vi "OLA.vi"() -> ()   [LabVIEW 2010]
doc: "This is the On-Line Analysis module (OLA).\nThis module receives events from the Target Event Builder (TEB) and processes them. The Q Curve is massaged, gains are divided out, the subtracted and poly subtracted signals are calculated, and an area measurement is made. These results are then sent to the Polarization Display Panel (PDP)."
panel:
  out "Bottom Charge":dbl format="%.6e"
  out "Top Charge":dbl format="%.6e"
  in  "Previous Event":i32
  in  "stop":bool
  out "RF Mod":i32
  out "RF Freq":dbl format="%.3f"
  out "Cal Const":dbl format="%.6f"
  out "Baseline":i32
  out "Raw Signal":dbl[](array[numeric]) format="%.4f"
  out "Event Number":i32
  out "Area":dbl format="%.6f"
  out "Polarization":dbl format="%.2f"
  out "PolySubtracted Signal":dbl[](array[numeric]) format="%.4f"
  out "Polyfit Curve":dbl[](array[numeric]) format="%.4f"
  out "Subtracted Signal":dbl[](array[numeric]) format="%.4f"
  out "Baseline Signal":dbl[](array[numeric]) format="%.6f"
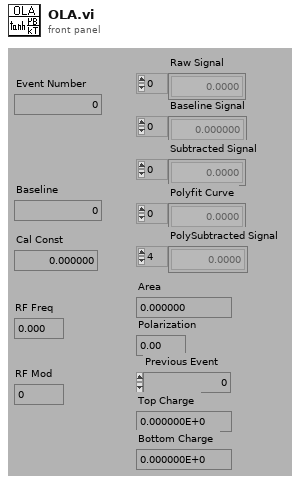
[diagram p1: front panel]
types:
  T1 = enum16{"No Message", "Bad Message", "ClearCharge", "Event=", "Address=", "Ping=", "Stop"}
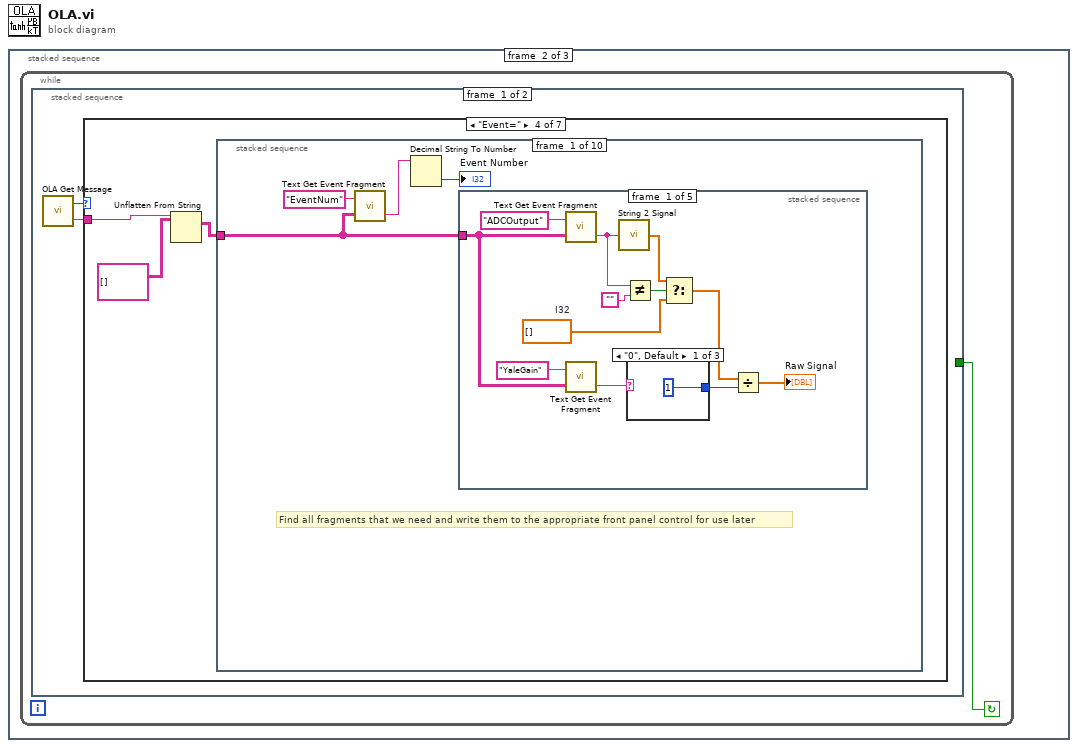
[diagram p0: block diagram]
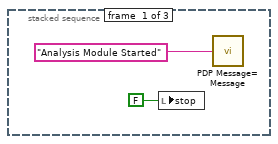
[diagram p2: hidden frame]
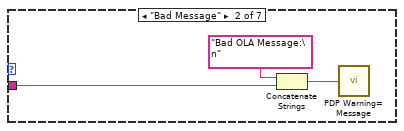
[diagram p4: hidden frame]
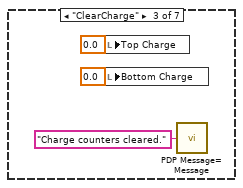
[diagram p5: hidden frame]
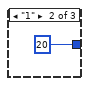
[diagram p6: hidden frame]
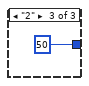
[diagram p7: hidden frame]
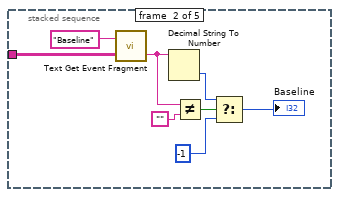
[diagram p8: hidden frame]
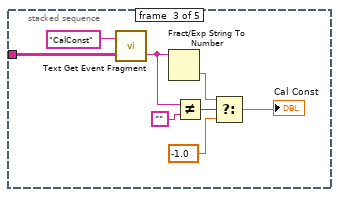
[diagram p9: hidden frame]
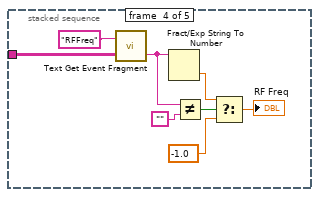
[diagram p10: hidden frame]
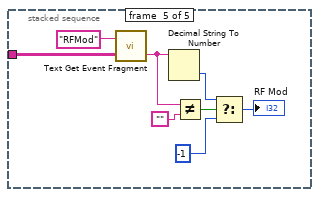
[diagram p11: hidden frame]
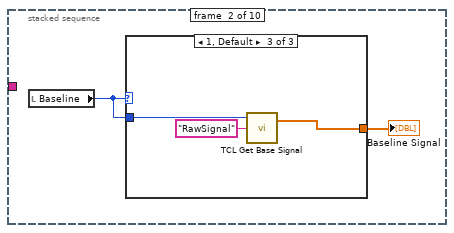
[diagram p12: hidden frame]
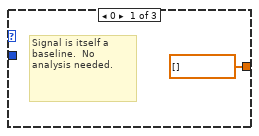
[diagram p13: hidden frame]
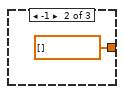
[diagram p14: hidden frame]
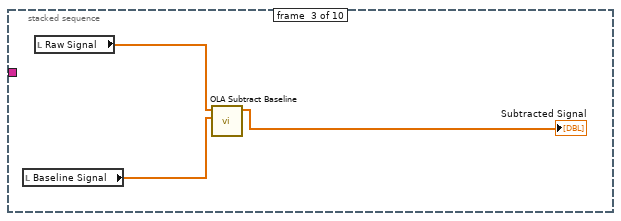
[diagram p15: hidden frame]
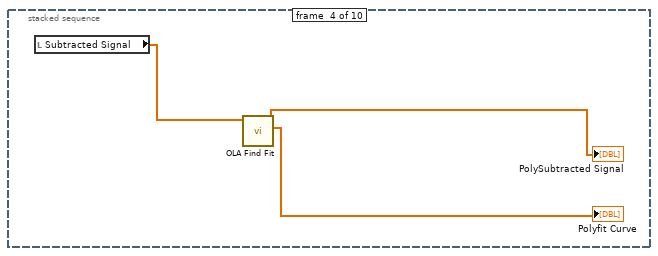
[diagram p16: hidden frame]
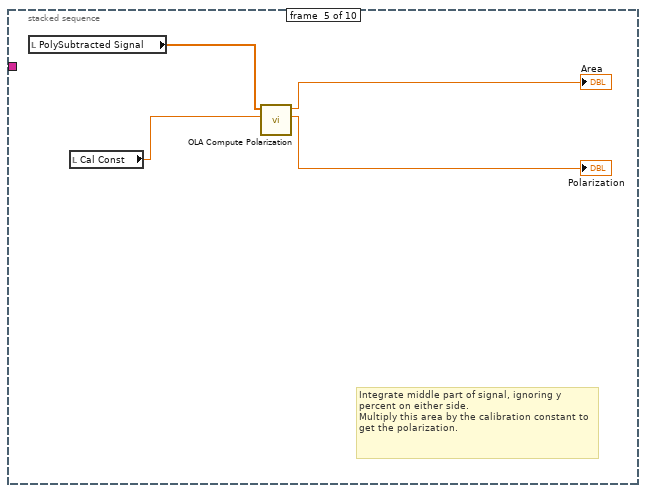
[diagram p17: hidden frame]
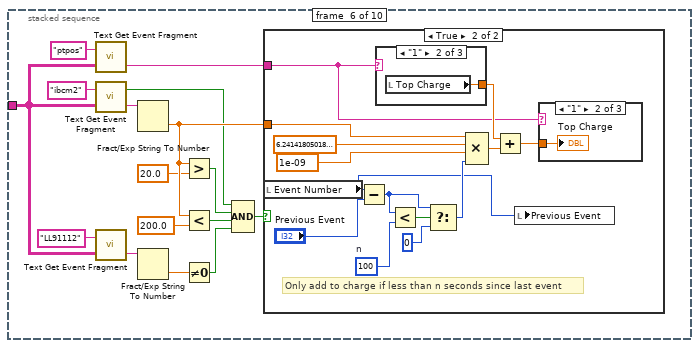
[diagram p18: hidden frame]
diagram:
  n1 = stacked-sequence {
    frame #0 {
      n2 = local write "stop"(FALSE ("stop")) -> ()
      n3 = call "PDP Message= Message.vi"("Message"="Analysis Module Started") -> ()
    }
    frame #1 {
      n4 = while {
        stop <- w3 continue-if-true
        n5 = stacked-sequence {
          tunnel: [_ w221] -> w3
          frame #0 {
            n6 = call "OLA Get Message.vi"() -> ("Text"=w5:string, "OLA Message Type"=w4:T1)
            n7 = case shown="\"Event=\"" w4 {
              tunnel: w5 -> [_ w8 _ w13 w213 w216 _]
              frame "No Message" {
              }
              frame "Bad Message" {
                n8 = Concatenate Strings("Bad OLA Message:\n", w8) -> (w6:string)
                n9 = call "PDP Warning= Message.vi"("Message"=w6) -> ()
              }
              frame "ClearCharge" {
                n10 = local write "Top Charge"(0.0 ("Top Charge")) -> ()
                n11 = local write "Bottom Charge"(0.0 ("Bottom Charge")) -> ()
                n12 = call "PDP Message= Message.vi"("Message"="Charge counters cleared.") -> ()
              }
              frame "Event=" {
                (unwired) FALSE
                n13 = Unflatten From String(type=string[][] [], binary string=w13) -> (value=w12:string[][])  [unwired: 3 in, 2 out]
                n14 = stacked-sequence {
                  tunnel: w12 -> [w15 _ _ _ _ w86 w119 w138 _ _]
                  frame #0 {
                    # "Find all fragments that we need and write them to the appropriate front panel control for use later"
                    n15 = call "Text Get Event Fragment.vi"("Event"=w15, "Fragment Type"="EventNum") -> ("Fragment"=w17:string)  [unwired: 1 out]
                    n16 = Decimal String To Number(string=w17) -> (number=→"Event Number":i32)  [unwired: 2 in, 1 out]
                    n17 = stacked-sequence {
                      tunnel: w15 -> [w24 w40 w48 w56 w64]
                      frame #0 {
                        w19 = dbl[] []  # I32
                        n18 = call "Text Get Event Fragment.vi"("Event"=w24, "Fragment Type"="ADCOutput") -> ("Fragment"=w29:string)  [unwired: 1 out]
                        n19 = call "Text Get Event Fragment.vi"("Event"=w24, "Fragment Type"="YaleGain") -> ("Fragment"=w23:string)  [unwired: 1 out]
                        n20 = call "String 2 Signal.vi"("String"=w29) -> ("Signal"=w26:dbl[])
                        n21 = Not Equal?(x=w29, y="") -> (x != y?=w28:bool)
                        n22 = case shown="\"0\", Default" w23 {
                          tunnel: [1 20 50] -> w22
                          frame "0", Default {
                          }
                          frame "1" {
                          }
                          frame "2" {
                          }
                        }
                        n23 = Select(t=w26, s=w28, f=w19) -> (s? t:f=w21:dbl[])
                        n24 = Divide(x=w21, y=w22) -> (x/y=→"Raw Signal":dbl[])
                      }
                      frame #1 {
                        n25 = call "Text Get Event Fragment.vi"("Event"=w40, "Fragment Type"="Baseline") -> ("Fragment"=w35:string)  [unwired: 1 out]
                        n26 = Decimal String To Number(string=w35) -> (number=w38:i32)  [unwired: 2 in, 1 out]
                        n27 = Not Equal?(x=w35, y="") -> (x != y?=w37:bool)
                        n28 = Select(t=w38, s=w37, f=-1) -> (s? t:f=→"Baseline":i32)
                      }
                      frame #2 {
                        n29 = call "Text Get Event Fragment.vi"("Event"=w48, "Fragment Type"="CalConst") -> ("Fragment"=w43:string)  [unwired: 1 out]
                        n30 = Fract/Exp String To Number(string=w43) -> (number=w46:dbl)  [unwired: 3 in, 1 out]
                        n31 = Not Equal?(x=w43, y="") -> (x != y?=w45:bool)
                        n32 = Select(t=w46, s=w45, f=-1.0) -> (s? t:f=→"Cal Const":dbl)
                      }
                      frame #3 {
                        n33 = call "Text Get Event Fragment.vi"("Event"=w56, "Fragment Type"="RFFreq") -> ("Fragment"=w51:string)  [unwired: 1 out]
                        n34 = Fract/Exp String To Number(string=w51) -> (number=w54:dbl)  [unwired: 3 in, 1 out]
                        n35 = Not Equal?(x=w51, y="") -> (x != y?=w53:bool)
                        n36 = Select(t=w54, s=w53, f=-1.0) -> (s? t:f=→"RF Freq":dbl)
                      }
                      frame #4 {
                        n37 = call "Text Get Event Fragment.vi"("Event"=w64, "Fragment Type"="RFMod") -> ("Fragment"=w59:string)  [unwired: 1 out]
                        n38 = Decimal String To Number(string=w59) -> (number=w62:i32)  [unwired: 2 in, 1 out]
                        n39 = Not Equal?(x=w59, y="") -> (x != y?=w61:bool)
                        n40 = Select(t=w62, s=w61, f=-1) -> (s? t:f=→"RF Mod":i32)
                      }
                    }
                  }
                  frame #1 {
                    n41 = local read "Baseline"() -> (w67:i32)
                    n42 = case shown="1, Default" w67 {
                      tunnel: w67 -> [_ _ w72]
                      tunnel: [dbl[] [] ("Baseline") dbl[] [] ("Baseline") w71] -> w66
                      frame 0 {
                        # "Signal is itself a baseline.  No analysis needed."
                      }
                      frame -1 {
                      }
                      frame 1, Default {
                        n43 = call "TCL Get Base Signal.vi"("signal name"="RawSignal", "event number"=w72) -> ("signal"=w71:dbl[])  [unwired: 1 in, 1 out]
                      }
                    }
                    "Baseline Signal" <- w66
                  }
                  frame #2 {
                    n44 = local read "Baseline Signal"() -> (w74:dbl[])
                    n45 = local read "Raw Signal"() -> (w75:dbl[])
                    n46 = call "OLA Subtract Baseline.vi"("baseline"=w74, "raw"=w75) -> ("subtracted"=→"Subtracted Signal":dbl[])  [unwired: 9 in]
                  }
                  frame #3 {
                    n47 = local read "Subtracted Signal"() -> (w78:dbl[])
                    n48 = call "OLA Find Fit.vi"("signal"=w78) -> ("fit"=→"Polyfit Curve":dbl[], "subtracted"=→"PolySubtracted Signal":dbl[])  [unwired: 8 in, 1 out]
                  }
                  frame #4 {
                    # "Integrate middle part of signal, ignoring y percent on either side.\nMultiply this area by the calibration constant to get the polarization."
                    n49 = local read "PolySubtracted Signal"() -> (w82:dbl[])
                    n50 = local read "Cal Const"() -> (w81:dbl)
                    n51 = call "OLA Compute Polarization.vi"("cal"=w81, "signal"=w82) -> ("polarization"=→"Polarization":dbl, "area"=→"Area":dbl)  [unwired: 8 in]
                  }
                  frame #5 {
                    n52 = call "Text Get Event Fragment.vi"("Event"=w86, "Fragment Type"="ptpos") -> ("Fragment"=w84:string)  [unwired: 1 out]
                    n53 = call "Text Get Event Fragment.vi"("Event"=w86, "Fragment Type"="ibcm2") -> ("Fragment"=w95:string, "Found"=w83:bool)
                    n54 = call "Text Get Event Fragment.vi"("Event"=w86, "Fragment Type"="LL91112") -> ("Fragment"=w97:string)  [unwired: 1 out]
                    n55 = Fract/Exp String To Number(string=w95) -> (number=w94:dbl)  [unwired: 3 in, 1 out]
                    n56 = Fract/Exp String To Number(string=w97) -> (number=w96:dbl)  [unwired: 3 in, 1 out]
                    n57 = Greater?(x=w94, y=20.0) -> (0:w89:bool)
                    n58 = Less?(x=w94, y=200.0) -> (x < y?=w91:bool)
                    n59 = Not Equal To 0?(x=w96) -> (x != 0?=w90:bool)
                    n60 = Compound Arithmetic op=AND(w83, w89, w91, w90) -> (w88:bool)
                    n61 = case shown="True" w88 {
                      tunnel: w94 -> [_ w109]
                      tunnel: w84 -> [_ w100]
                      frame False {
                      }
                      frame True {
                        w108 = 100  # n
                        # "Only add to charge if less than n seconds since last event"
                        n62 = local read "Event Number"() -> (w99:i32)
                        n63 = Subtract(x=w99, y="Previous Event") -> (x-y=w105:i32)
                        n64 = case shown="\"1\"" w100 {
                          tunnel: [0.0 w116 w117] -> w102
                          frame "0", Default {
                          }
                          frame "1" {
                            n65 = local read "Top Charge"() -> (w116:dbl)
                          }
                          frame "2" {
                            n66 = local read "Bottom Charge"() -> (w117:dbl)
                          }
                        }
                        n67 = Less?(x=w105, y=w108) -> (x < y?=w106:bool)
                        n68 = Select(t=w105, s=w106, f=0) -> (s? t:f=w103:i32)
                        n69 = Compound Arithmetic op=MULTIPLY(w109, 6.241418050181001e+18, 1e-09 ("Input"), w103) -> (w107:dbl)
                        n70 = Add(x=w102, y=w107) -> (x+y=w101:dbl)
                        n71 = local write "Previous Event"(w99) -> ()
                        n72 = case shown="\"1\"" w100 {
                          tunnel: w101 -> [_ w113 w114]
                          frame "0", Default {
                          }
                          frame "1" {
                            "Top Charge" <- w113
                          }
                          frame "2" {
                            "Bottom Charge" <- w114
                          }
                        }
                      }
                    }
                  }
                  frame #6 {
                    n73 = call "Text Get Event Fragment.vi"("Event"=w119, "Fragment Type"="He4Temp") -> ("Found"=w118:bool)  [unwired: 1 out]
                    n74 = case shown="False" w118 {
                      tunnel: w119 -> [w127 _]
                      frame False {
                        n75 = call "Text Get Event Fragment.vi"("Event"=w127, "Fragment Type"="He4Press") -> ("Fragment"=w135:string)  [unwired: 1 out]
                        n76 = call "Text Get Event Fragment.vi"("Event"=w127, "Fragment Type"="He4Range") -> ("Fragment"=w126:string)  [unwired: 1 out]
                        n77 = Fract/Exp String To Number(string=w135) -> (number=w121:dbl)  [unwired: 3 in, 1 out]
                        n78 = Fract/Exp String To Number(string=w126) -> (number=w125:dbl)  [unwired: 3 in, 1 out]
                        n79 = expression code="10**(-x+2)"(w125) -> (w124:dbl)
                        n80 = Multiply(x=w121, y=w124) -> (x*y=w122:dbl)
                        n81 = call "TTM 4He Press to Temp.vi"("4He Vapor Pressure (torr)"=w122) -> ("4He Temp (K)"=w123:dbl)
                        n82 = Number To Exponential String(number=w123) -> (E-format string=w133:string)  [unwired: 3 in]
                        n83 = local read "Event Number"() -> (w130:i32)
                        n84 = Build Array("He4Temp", w133) -> (w129:string[])
                        n85 = Build Array(w129) -> (w131:string[][])
                        n86 = call "TEB EventFrag= Message.vi"("Event Fragment(s)"=w131, "Event Number"=w130) -> ()
                      }
                      frame True {
                      }
                    }
                  }
                  frame #7 {
                    n87 = call "Text Get Event Fragment.vi"("Event"=w138, "Fragment Type"="HPFreq") -> ("Fragment"=w136:string, "Found"=w137:bool)
                    n88 = case shown="True" w137 {
                      tunnel: w138 -> [w141 w159]
                      tunnel: w136 -> [_ w156]
                      frame False {
                        n89 = call "Text Get Event Fragment.vi"("Event"=w141, "Fragment Type"="EIPFreq") -> ("Fragment"=w140:string)  [unwired: 1 out]
                        n90 = local read "Event Number"() -> (w143:i32)
                        n91 = Build Array("uWaveFreq", w140) -> (w142:string[])
                        n92 = Build Array(w142) -> (w144:string[][])
                        n93 = call "TEB EventFrag= Message.vi"("Event Fragment(s)"=w144, "Event Number"=w143) -> ()
                      }
                      frame True {
                        n94 = call "Text Get Event Fragment.vi"("Event"=w159, "Fragment Type"="EIPFreq") -> ("Fragment"=w158:string)  [unwired: 1 out]
                        n95 = Fract/Exp String To Number(string=w156) -> (number=w149:dbl)  [unwired: 3 in, 1 out]
                        n96 = Fract/Exp String To Number(string=w158) -> (number=w157:dbl)  [unwired: 3 in, 1 out]
                        n97 = Multiply(x=w157, y=2) -> (x*y=w155:dbl)
                        n98 = Add(x=w149, y=w155) -> (x+y=w154:dbl)
                        n99 = Equal To 0?(x=w149) -> (x = 0?=w148:bool)
                        n100 = Number To Fractional String(number=w154, precision (6)=i16 3) -> (F-format string=w150:string)  [unwired: 2 in]
                        n101 = Select(t="0", s=w148, f=w150) -> (s? t:f=w151:string)
                        n102 = local read "Event Number"() -> (w161:i32)
                        n103 = Build Array("uWaveFreq", w151) -> (w160:string[])
                        n104 = Build Array(w160) -> (w162:string[][])
                        n105 = call "TEB EventFrag= Message.vi"("Event Fragment(s)"=w162, "Event Number"=w161) -> ()
                      }
                    }
                  }
                  frame #8 {
                    w167 = string[] [] ("Array Constant")
                    # "Ship all results off to the event builder."
                    n106 = local read "PolySubtracted Signal"() -> (w165:dbl[])
                    n107 = local read "Bottom Charge"() -> (w177:dbl)
                    n108 = local read "Subtracted Signal"() -> (w202:dbl[])
                    n109 = local read "Polyfit Curve"() -> (w201:dbl[])
                    n110 = local read "Polarization"() -> (w188:dbl)
                    n111 = local read "Baseline Signal"() -> (w207:dbl[])
                    n112 = local read "Top Charge"() -> (w178:dbl)
                    n113 = local read "Raw Signal"() -> (w185:dbl[])
                    n114 = local read "Area"() -> (w196:dbl)
                    n115 = Array Size(array=w165) -> (size(s)=w166:i32)
                    n116 = Equal To 0?(x=w166) -> (x = 0?=w168:bool)
                    n117 = call "Signal 2 String.vi"("Signal"=w185) -> ("String"=w186:string)
                    n118 = call "Signal 2 String.vi"("Signal"=w207) -> ("String"=w206:string)
                    n119 = call "Signal 2 String.vi"("Signal"=w202) -> ("String"=w203:string)
                    n120 = call "Signal 2 String.vi"("Signal"=w201) -> ("String"=w200:string)
                    n121 = call "Signal 2 String.vi"("Signal"=w165) -> ("String"=w197:string)
                    n122 = Number To Exponential String(number=w178) -> (E-format string=w180:string)  [unwired: 3 in]
                    n123 = Number To Exponential String(number=w177) -> (E-format string=w175:string)  [unwired: 3 in]
                    n124 = Number To Exponential String(number=w188) -> (E-format string=w189:string)  [unwired: 3 in]
                    n125 = Number To Exponential String(number=w196) -> (E-format string=w195:string)  [unwired: 3 in]
                    n126 = Build Array("RawSignal", w186) -> (w184:string[])
                    n127 = Build Array("BaseSignal", w206) -> (w183:string[])
                    n128 = Build Array("SubSignal", w203) -> (w182:string[])
                    n129 = Build Array("PolyCurve", w200) -> (w181:string[])
                    n130 = Build Array("PolySignal", w197) -> (w193:string[])
                    n131 = Build Array("TopCharge", w180) -> (w174:string[])
                    n132 = Build Array("BottomCharge", w175) -> (w173:string[])
                    n133 = Build Array("Polarization", w189) -> (w172:string[])
                    n134 = Build Array("Area", w195) -> (w171:string[])
                    n135 = Select(t=w167, s=w168, f=w172) -> (s? t:f=w169:string[])
                    n136 = Select(t=w167, s=w168, f=w171) -> (s? t:f=w170:string[])
                    n137 = local read "Event Number"() -> (w191:i32)
                    n138 = Build Array(w184, w183, w182, w181, w193, w174, w173, w169, w170) -> (w192:string[][])
                    n139 = call "TEB EventFrag= Message.vi"("Event Fragment(s)"=w192, "Event Number"=w191) -> ()
                  }
                  frame #9 {
                    # "Tell event builder we're done processing this event."
                    n140 = local read "Event Number"() -> (w209:i32)
                    n141 = call "TEB Processed= Message.vi"("Module Name"="OLA", "Event Number"=w209) -> ()
                  }
                }
              }
              frame "Address=" {
                n142 = Scan From String(format string="%s,%[.0-9]:%d" ("Format String"), input string=w213) -> (output 1=w211:string, output 2=w212:string, output 3=w210:i32)  [unwired: 5 in, 3 out]
                n143 = call "Message Set Module Address.vi"("Port"=w210, "Address"=w212, "Module"=w211) -> ()
              }
              frame "Ping=" {
                n144 = Get Date/Time In Seconds() -> (seconds since 1Jan1904=w215:timestamp)
                n145 = To Double Precision Float(number=w215) -> (double precision float=w218:dbl)
                n146 = Format Into String(format string="PingResponse=OLA,%.0f", w218) -> (resulting string=w217:string)  [unwired: 2 in, 1 out]
                n147 = call "Message Send.vi"("Message"=w217, "Destination"=w216) -> ()
              }
              frame "Stop" {
                n148 = local write "stop"(TRUE ("stop")) -> ()
              }
            }
          }
          frame #1 {
            n149 = Not(x="stop") -> (.not. x?=w221:bool)
          }
        }
      }
    }
    frame #2 {
      n150 = local write "stop"(FALSE ("stop")) -> ()
      n151 = call "PDP Message= Message.vi"("Message"="OLA Module Stopped") -> ()
    }
  }
